vi "readConfig.vi"(8 "error in (no error)":errorcluster, 9 "config":string, 10 "deviceName":string, 11 "Dio64FileReader in":refnum<class "Dio64FileReader.lvclass">) -> (0 "error out":errorcluster, 3 "Dio64FileReader out":refnum<class "Dio64FileReader.lvclass">)   [LabVIEW 2011, in "Tools.lvlib" / "Filing.lvlib" / "Dio64FileReader.lvclass"]
uses:
  Dio64FileReader.lvclass
  Hal/Channels/Digital/DigitalOutput.lvclass
  Dio64FileReader.lvclass/Dio64FileReader.ctl
  FileReader.lvclass
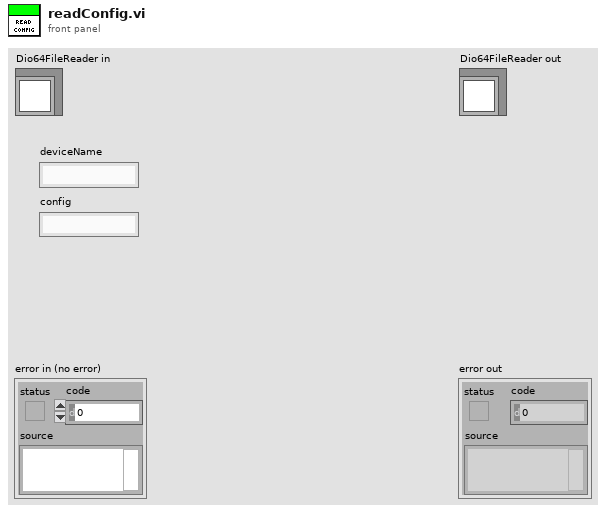
[diagram p1: front panel]
types:
  T1 = cluster{"Master Clock source":string, "Master Clock rate":dbl, "Start trigger line":string, "Scan rate":dbl, "Stop trigger line":string, "Sample Number":dbl}
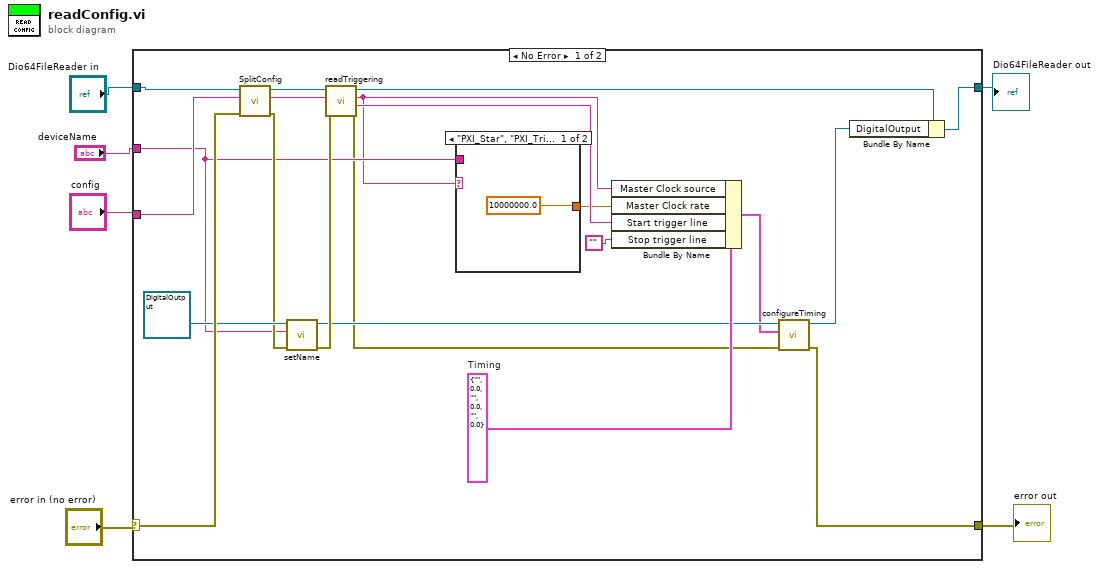
[diagram p0: block diagram]
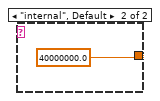
[diagram p2: hidden frame]
diagram:
  n1 = case shown="No Error" "error in (no error)" {
    selector: "error in (no error)" -> [w26 w30]
    tunnel: "Dio64FileReader in" -> [w27 w31]
    tunnel: [w20 w31] -> w5
    tunnel: [w7 w30] -> w4
    tunnel: "config" -> [w25 _]
    tunnel: "deviceName" -> [w16 _]
    frame No Error {
      w13 = T1 {"Master Clock source"="", "Master Clock rate"=0.0, "Start trigger line"="", "Scan rate"=0.0, "Stop trigger line"="", "Sample Number"=0.0}  # Timing
      n2 = call "SplitConfig.vi"("error in (no error)"=w26, "Config"=w25, "FileReader in"=w27) -> ("error out"=w18:errorcluster, "triggering"=w23:string, "FileReader out"=w24:refnum<class "Dio64FileReader.lvclass">)  [unwired: 4 in, 2 out]
      n3 = call-dynamic "setName.vi"("error in (no error)"=w18, "name"=w16, "DigitalOutput.lvclass in"=refnum<class "DigitalOutput.lvclass"> refnum ("DigitalOutput")) -> ("error out"=w17:errorcluster, "DigitalOutput.lvclass out"=w11:refnum<class "DigitalOutput.lvclass">)  [unwired: 7 in]
      n4 = call-dynamic "readTriggering.vi"("error in (no error)"=w17, "triggering"=w23, "FileReader in"=w24) -> ("error out"=w10:errorcluster, "start trigger line"=w22:string, "clock source"=w15:string, "FileReader out"=w21:refnum<class "Dio64FileReader.lvclass">)  [unwired: 5 in]
      n5 = case shown="\"PXI_Star\", \"PXI_Trig_00\", \"PXI_Trig_01\", \"PXI_Trig_02\", \"PXI_Trig_03\", \"PXI_Trig_04\", \"PXI_Trig_05\", \"PXI_Trig_06\", \"PXI_Trig_07\"" w15 {
        tunnel: [10000000.0 40000000.0] -> w14
        tunnel: w16 -> [_ _]
        frame "PXI_Star", "PXI_Trig_00", "PXI_Trig_01", "PXI_Trig_02", "PXI_Trig_03", "PXI_Trig_04", "PXI_Trig_05", "PXI_Trig_06", "PXI_Trig_07" {
        }
        frame "internal", Default {
        }
      }
      n6 = Bundle By Name(cluster=w13, "Master Clock source"=w15, "Master Clock rate"=w14, "Start trigger line"=w22, "Stop trigger line"="") -> (w9:T1)
      n7 = call-dynamic "configureTiming.vi"("error in (no error)"=w10, "Timing"=w9, "DigitalOutput in"=w11) -> ("error out"=w7:errorcluster, "DigitalOutput out"=w8:refnum<class "DigitalOutput.lvclass">)  [unwired: 7 in]
      n8 = Bundle By Name(cluster=w21, "DigitalOutput"=w8) -> (w20:refnum<class "Dio64FileReader.lvclass">)
    }
    frame Error {
    }
  }
  "error out" <- w4
  "Dio64FileReader out" <- w5
